vi "Euler Project Problem 1 Solution (3).vi"() -> ()   [LabVIEW 2017]
panel:
  out "Total":i32
  in  "Multiple 2":i32=5
  in  "Multiple 1":i32=3
  # "Problem description from the project Euler Website:\n\nAdd all the natural numbers below one thousand that are multiples of 3 or 5."
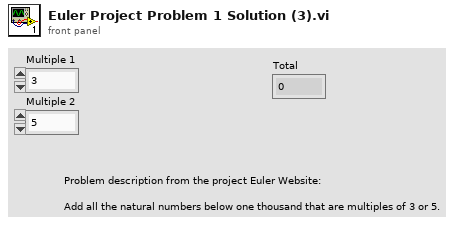
[diagram p1: front panel]
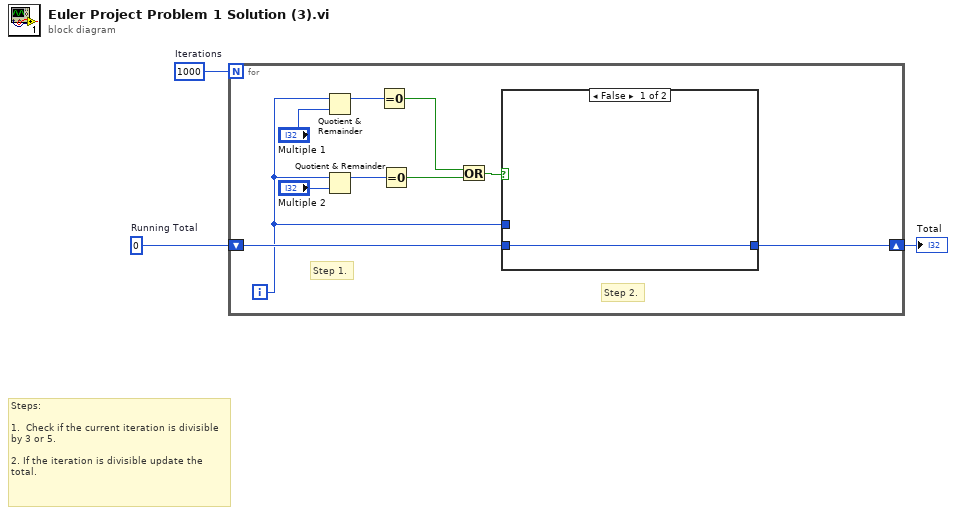
[diagram p0: block diagram]
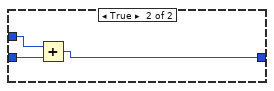
[diagram p2: hidden frame]
diagram:
  w2 = 0  # Running Total
  w3 = 1000  # Iterations
  # "Steps:\n\n1.  Check if the current iteration is divisible by 3 or 5.\n\n2. If the iteration is divisible update the total."
  n1 = for {
    N: w3 -> [_]
    shift-right: [w4] -> w1
    shift-left: w2 -> [w6]
    i -> [w5]
    # "Step 2."
    # "Step 1."
    n2 = Quotient & Remainder(x=w5, y="Multiple 1") -> (x-y*floor(x/y)=w11:i32)  [unwired: 1 out]
    n3 = Quotient & Remainder(x=w5, y="Multiple 2") -> (x-y*floor(x/y)=w10:i32)  [unwired: 1 out]
    n4 = Equal To 0?(x=w11) -> (x = 0?=w9:bool)
    n5 = Equal To 0?(x=w10) -> (x = 0?=w8:bool)
    n6 = Or(x=w9, y=w8) -> (x .or. y?=w7:bool)
    n7 = case shown="False" w7 {
      tunnel: w6 -> [w14 w16]
      tunnel: w5 -> [_ w17]
      tunnel: [w14 w15] -> w4
      frame False {
      }
      frame True {
        n8 = Add(x=w17, y=w16) -> (x+y=w15:i32)
      }
    }
  }
  "Total" <- w1
